vi "Last_check.vi"(11 "in_Array":dbl[][](array[numeric])) -> (3 "out Array":dbl[][](array[numeric]))   [LabVIEW 2014]
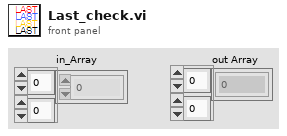
[diagram p1: front panel]
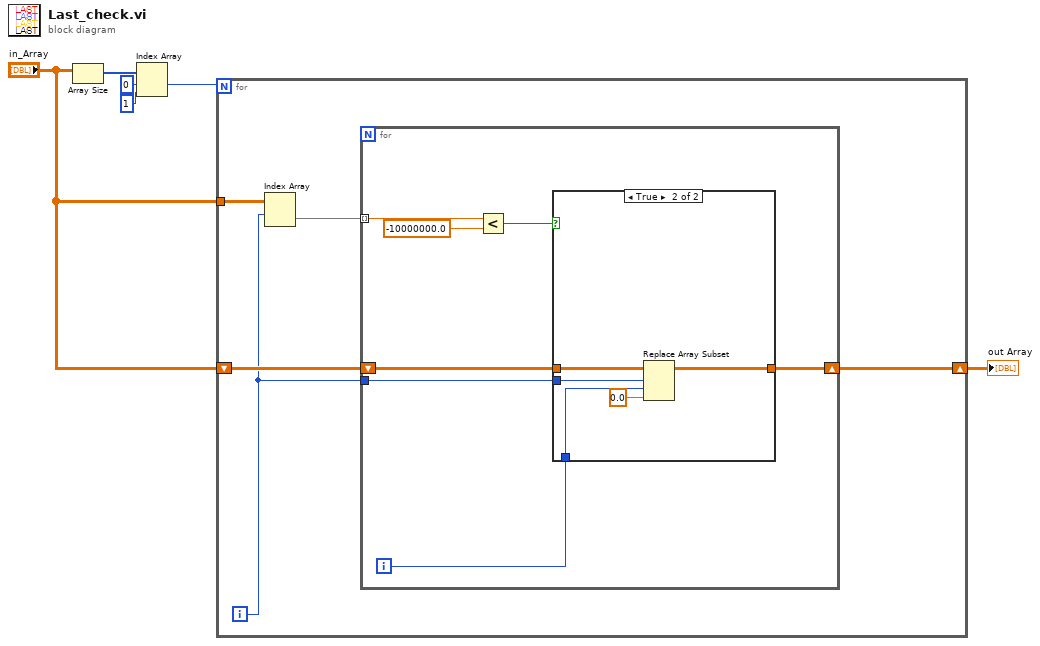
[diagram p0: block diagram]
diagram:
  n1 = Array Size(array="in_Array") -> (size(s)=w6:i32[])
  n2 = Index Array(array=w6, index #1=0 ("index"), index #2=1 ("index")) -> (element #1=w3:i32)  [unwired: 1 out]
  n3 = for {
    N: w3 -> [_]
    tunnel: "in_Array" -> [w11]
    shift-right: [w8] -> w1
    shift-left: "in_Array" -> [w9]
    i -> [w7]
    n4 = Index Array(array=w11, index (row)=w7) -> (element=w10:dbl[])  [unwired: 1 in]
    n5 = for {
      tunnel: w10 -> [w18] mode=indexing
      shift-right: [w14] -> w8
      shift-left: w9 -> [w15]
      tunnel: w7 -> [w13]
      i -> [w12]
      n6 = Less?(x=w18, y=-10000000.0) -> (x < y?=w16:bool)
      n7 = case shown="True" w16 {
        tunnel: w15 -> [w19 w24]
        tunnel: [w19 w23] -> w14
        tunnel: w13 -> [_ w22]
        tunnel: w12 -> [_ w21]
        frame False {
        }
        frame True {
          n8 = Replace Array Subset(array=w24, new element=0.0 ("new element/subarray"), index (row)=w22, index (col)=w21) -> (w23:dbl[][])
        }
      }
    }
  }
  "out Array" <- w1
